vi "CloseDataClassReference.vi"(8 "error in (no error)":errorcluster, 11 "DataClassNotifierIn":refnum<notifier>) -> (0 "error out":errorcluster, 3 "Data out":refnum<class "Data.lvclass">)   [LabVIEW 2013, in "Data.lvclass"]
uses:
  Data.lvclass
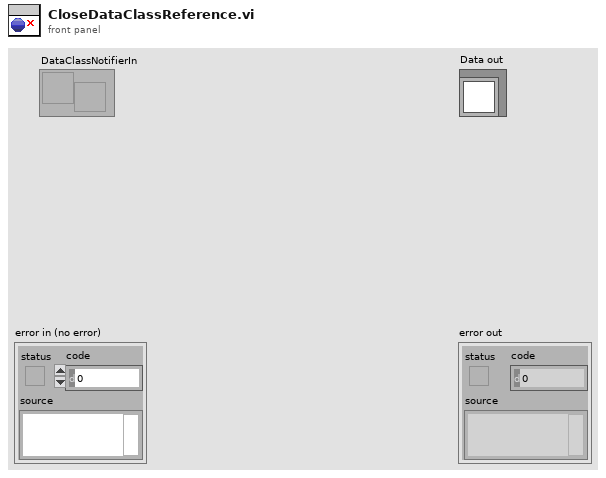
[diagram p1: front panel]
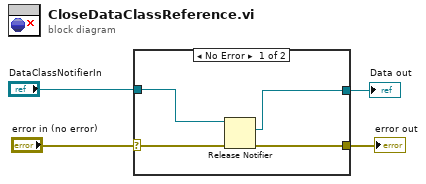
[diagram p0: block diagram]
diagram:
  n1 = case shown="No Error" "error in (no error)" {
    selector: "error in (no error)" -> [w8 w9]
    tunnel: [w7 w9] -> w3
    tunnel: "DataClassNotifierIn" -> [w6 _]
    tunnel: [w5 _] -> w1
    frame No Error {
      n2 = Release Notifier(notifier=w6, error in (no error)=w8) -> (last notification=w5:refnum<class "Data.lvclass">, error out=w7:errorcluster)  [unwired: 1 in, 1 out]
    }
    frame Error {
    }
  }
  "error out" <- w3
  "Data out" <- w1
